vi "check for new image.vi"(3 "Acq Img":T1, 4 "Buffer":T1, 5 "Downloaded image":T1) -> (0 "Error code -1074396074 i.e. image size diff.":bool, 1 "Image ok":bool, 2 "Image Out":T1)   [LabVIEW 2013]
uses:
  <vilib>/vision/Image Controls.llb/IMAQ Image.ctl
  <vilib>/vision/NI_Vision_Development_Module.lvlib
panel:
  out "error out 4":errorcluster
  out "x = y?":bool
  out "error out 3":errorcluster
  out "error out 2":errorcluster
  out "error out":errorcluster
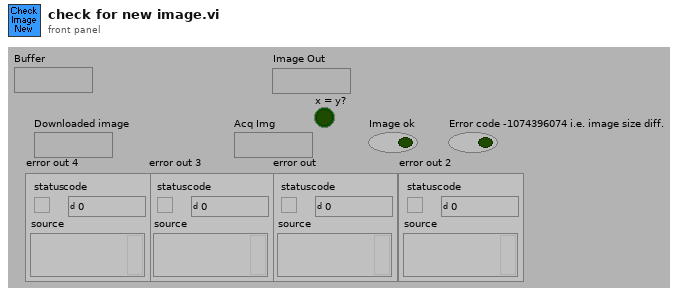
[diagram p1: front panel]
types:
  T1 = typedef "IMAQ Image.ctl" = refnum<image>
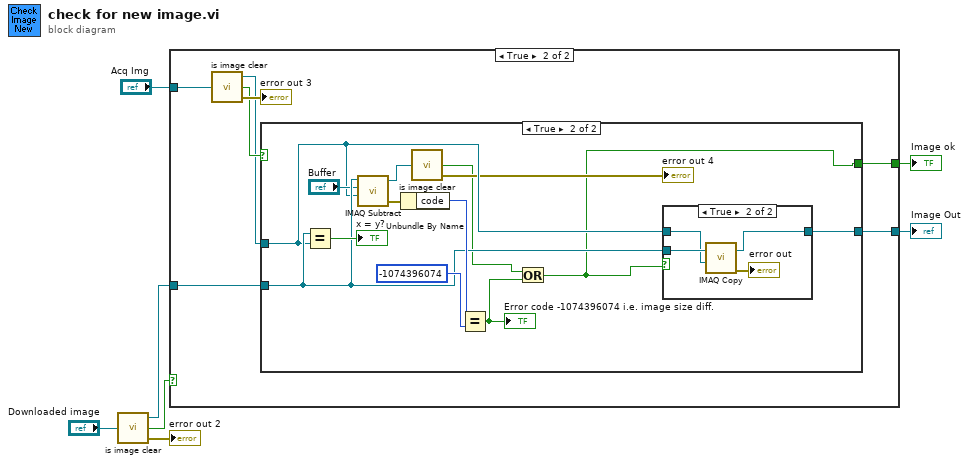
[diagram p0: block diagram]
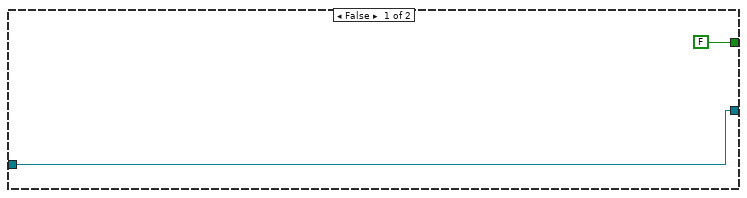
[diagram p2: hidden frame]
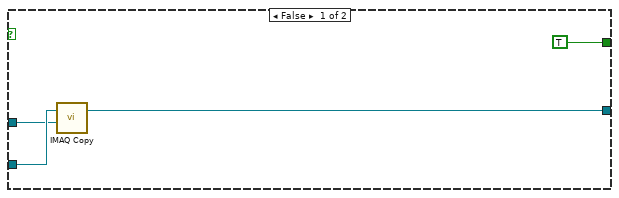
[diagram p3: hidden frame]
diagram:
  n1 = call "is image clear.vi"("Input image"="Downloaded image") -> ("Image Out"=w1:T1, "Image ok"=w6:bool, "error out"=→"error out 2":errorcluster)
  n2 = case shown="True" w6 {
    tunnel: [FALSE ("Image ok") w10] -> w5
    tunnel: "Acq Img" -> [_ w13]
    tunnel: w1 -> [w8 w14]
    tunnel: [w8 w11] -> w3
    frame False {
    }
    frame True {
      n3 = call "is image clear.vi"("Input image"=w13) -> ("Image Out"=w12:T1, "Image ok"=w15:bool, "error out"=→"error out 3":errorcluster)
      n4 = case shown="True" w15 {
        tunnel: w14 -> [w20 w30]
        tunnel: w12 -> [w19 w26]
        tunnel: [w18 w27] -> w11
        tunnel: [TRUE ("Image ok") w21] -> w10
        frame False {
          n5 = call "IMAQ Copy"("Image Dst"=w19, "Image Src"=w20) -> ("Image Dst Out"=w18:T1)  [unwired: 4 in, 1 out]
        }
        frame True {
          n6 = Equal?(x=w30, y=w26) -> (x = y?=→"x = y?":bool)
          n7 = call "IMAQ Subtract"("Image Src A"=w30, "Image Dst"="Buffer", "Image Src B"=w26) -> ("Image Dst Out"=w28:T1, "error out"=w25:errorcluster)  [unwired: 4 in]
          n8 = Unbundle By Name(w25) -> ("code"=w33:i32)
          n9 = call "is image clear.vi"("Input image"=w28) -> ("Image ok"=w23:bool, "error out"=→"error out 4":errorcluster)  [unwired: 1 out]
          n10 = Equal?(x=w33, y=-1074396074 ("code")) -> (x = y?=w22:bool)
          "Error code -1074396074 i.e. image size diff." <- w22
          n11 = Or(x=w23, y=w22) -> (x .or. y?=w21:bool)
          n12 = case shown="True" w21 {
            tunnel: w30 -> [_ w38]
            tunnel: [w34 w37] -> w27
            tunnel: w26 -> [w34 w35]
            frame False {
            }
            frame True {
              n13 = call "IMAQ Copy"("Image Dst"=w35, "Image Src"=w38) -> ("error out"=→"error out":errorcluster, "Image Dst Out"=w37:T1)  [unwired: 4 in]
            }
          }
        }
      }
    }
  }
  "Image ok" <- w5
  "Image Out" <- w3
